vi "CAN_COM.vi"() -> ()   [LabVIEW 2016]
uses:
  <vilib>/Platform/TimedLoop/XDataNode/timing_clust.ctl
  <vilib>/Platform/TimedLoop/XDataNode/nitl_modes.ctl
  <vilib>/Platform/TimedLoop/XDataNode/wakeup.ctl
  <vilib>/platform/TimedLoop/XDataNode/XDataNode.xnode
  <vilib>/Platform/TimedLoop/XDataNode/XDNodeRunTimeDep.lvlib
panel:
  out "MOD_6":bool
  out "MOD_1":bool
  in  "UNLOCK_LEVEL":bool
  in  "Stop RT":bool
  in  "Transmit Frame":T1={"timestamp high"=0, "timestamp low"=0, "identifier"=18, "type"=enum."Data Frame", "info A"=0, "info B"=0, "data length"=8, "data"=[0, 0, 0, 0, 0, 0, 0, 0]} {"identifier" format="%x"; "data" format="%.0x"}
  out "Total Received":u32
  out "Recent Receive":T2={"timestamp high"=0, "timestamp low"=0, "identifier"=0, "type"=enum."Data Frame", "info A"=0, "info B"=0, "data length"=0, "data"=[0, 0, 0, 0, 0, 0, 0, 0]} {"identifier" format="%.0x"; "data" format="%.0x"}
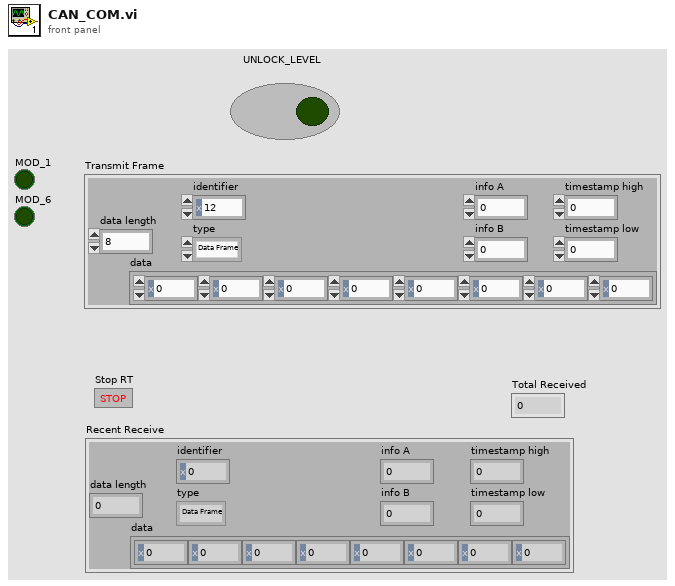
[diagram p1: front panel]
types:
  T1 = cluster{"timestamp high":u32, "timestamp low":u32, "identifier":u32, "type":enum8{"Data Frame", "Remote Frame", "(reserved)", "(reserved) ", "(reserved)  ", "(reserved)   ", "Bus Error", "Transceiver Fault"}, "info A":u8, "info B":u8, "data length":u8, "data":u32[]}
  T2 = cluster{"timestamp high":u32, "timestamp low":u32, "identifier":u32, "type":enum8{"Data Frame", "Remote Frame", "(reserved)", "(reserved) ", "(reserved)  ", "(reserved)   ", "Bus Error", "Transceiver Fault"}, "info A":u8, "info B":u8, "data length":u8, "data":u8[]}
  T3 = typedef "XDNodeRunTimeDep.lvlib/timing_clust.ctl" = cluster{"Expected End [f-1]":u64, "Actual End [f-1]":u64, "Finished Late? [f-1]":bool, "Expected End [i-1]":u64, "Actual End [i-1]":u64, "Finished Late? [i-1]":bool, "Expected Start [i]":u64, "Actual Start [i]":u64, "Expected Start [f]":u64, "Actual Start [f]":u64, "Source Name":string, "Structure Name":string, "Period":i64, "Deadline":i64, "Offset":i64, "Start":i64, "Priority":i32, "Timeout":i32, "Mode":T4, "Wakeup Reason":T5, "Error":errorcluster, "Source Type":string, "Secondary Source Type":string, "Global End Time":u64, "Global Start Time":u64, "Frame Duration":u64, "Iteration Duration":u64, "Assigned CPU":i32, "I/O Scan Engine Mode":u32}
  T4 = typedef "XDNodeRunTimeDep.lvlib/nitl_modes.ctl" = enum32{"No Change", "Process missed periods, maintain original phase", "Discard missed periods, maintain original phase", "Process missed periods, ignore original phase", "Discard missed periods, ignore original phase"}
  T5 = typedef "XDNodeRunTimeDep.lvlib/wakeup.ctl" = enum32{"Normal", "Aborted", "Asynchronous wakeup", "Timing source error", "Timed loop error", "Timeout"}
  T6 = enum8{"Data Frame", "Remote Frame", "(reserved)", "(reserved) ", "(reserved)  ", "(reserved)   ", "Bus Error", "Transceiver Fault"}
  T7 = cluster{"data[0]":u32, "data[1]":u32, "data[2]":u32, "data[3]":u32, "data[4]":u32, "data[5]":u32, "data[6]":u32, "data[7]":u32, "data[8]":u32}
  T8 = cluster{"data[0]":u8, "data[1]":u8, "data[2]":u8, "data[3]":u8, "data[4]":u8, "data[5]":u8, "data[6]":u8, "data[7]":u8, "data[8]":u8}
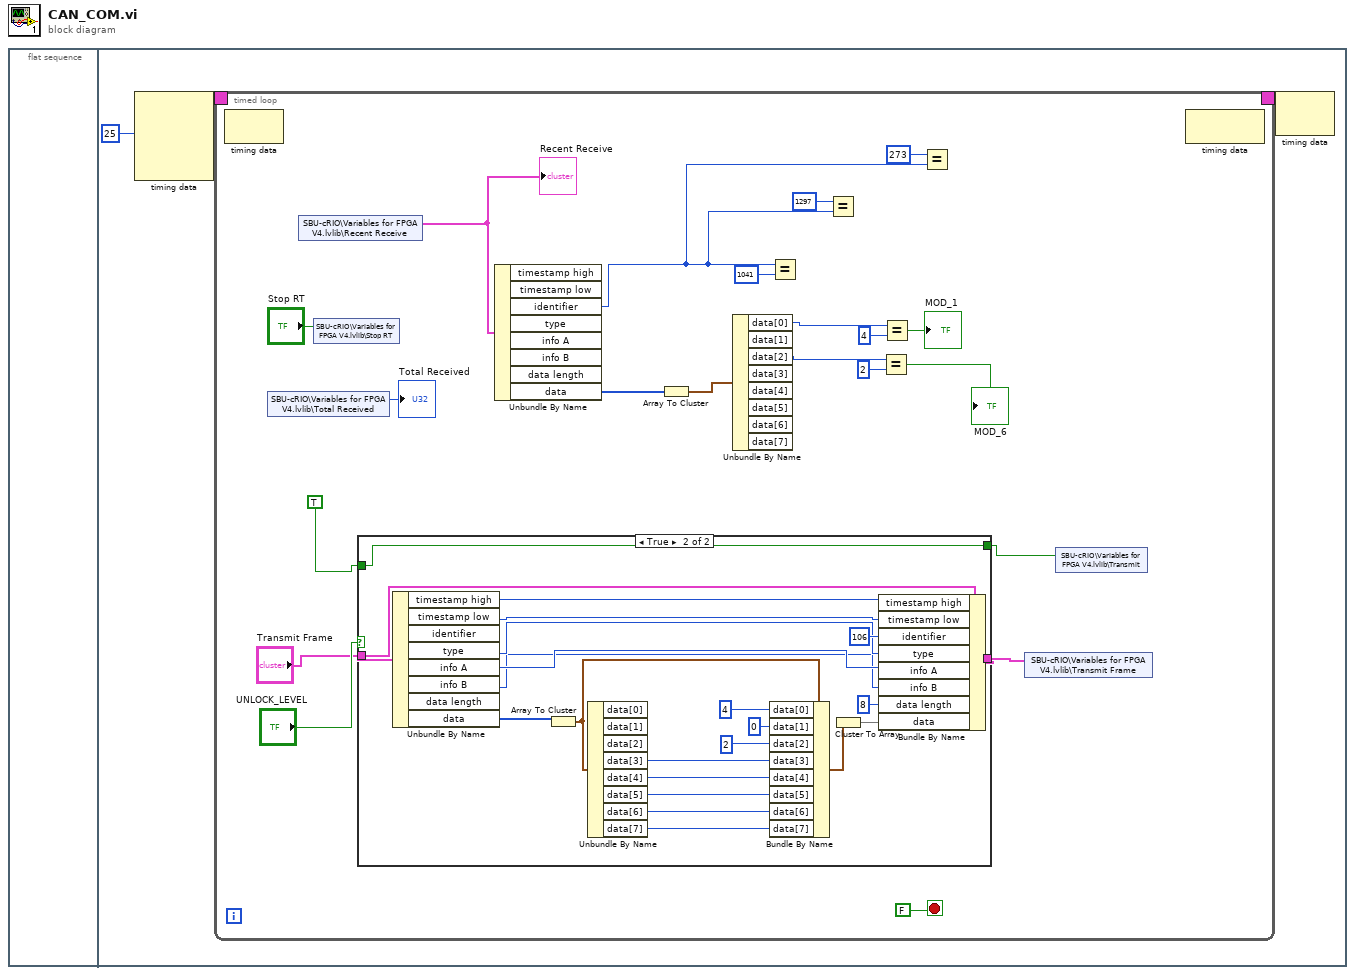
[diagram p0: block diagram]
diagram:
  n1 = flat-sequence {
    frame #0 {
    }
    frame #1 {
      n2 = node-c288(i64 25 ("Period")) -> (w3:T3)  [unwired: 3 in]
      n3 = timed-loop {
        timing: w3 -> [_]
        timing-out: [_] -> w2
        stop <- FALSE stop-if-true
        n4 = node-c288() -> ()  [unwired: 1 in, 1 out]
        n5 = shared-variable "SBU-cRIO\\Variables for FPGA V4.lvlib\\Total Received"() -> (→"Total Received":u32)  [unwired: 1 in, 1 out]
        n6 = shared-variable "SBU-cRIO\\Variables for FPGA V4.lvlib\\Recent Receive"() -> (w18:T2)  [unwired: 1 in, 1 out]
        "Recent Receive" <- w18
        n7 = shared-variable "SBU-cRIO\\Variables for FPGA V4.lvlib\\Stop RT"("Stop RT") -> ()  [unwired: 1 in, 1 out]
        n8 = case shown="True" "UNLOCK_LEVEL" {
          tunnel: "Transmit Frame" -> [w26 w38]
          tunnel: [w26 w39] -> w16
          tunnel: [w25 w34] -> w6
          tunnel: TRUE -> [w25 w34]
          frame False {
          }
          frame True {
            n9 = Unbundle By Name(w38) -> ("timestamp high"=w47:u32, "timestamp low"=w46:u32, "type"=w44:T6, "info A"=w43:u8, "info B"=w42:u8, "data"=w40:u32[])  [unwired: 2 out]
            n10 = Array To Cluster(array=w40) -> (cluster=w37:T7)
            n11 = Unbundle By Name(w37) -> ("data[3]"=w31:u32, "data[4]"=w30:u32, "data[5]"=w29:u32, "data[6]"=w28:u32, "data[7]"=w27:u32)  [unwired: 3 out]
            n12 = Bundle By Name(cluster=w37, "data[0]"=u32 4, "data[1]"=u32 0, "data[2]"=u32 2 ("identifier"), "data[3]"=w31, "data[4]"=w30, "data[5]"=w29, "data[6]"=w28, "data[7]"=w27) -> (w36:T7)
            n13 = Cluster To Array(cluster=w36) -> (array=w41:u32[])
            n14 = Bundle By Name(cluster=w38, "timestamp high"=w47, "timestamp low"=w46, "identifier"=u32 106, "type"=w44, "info A"=w43, "info B"=w42, "data length"=u8 8, "data"=w41) -> (w39:T1)
          }
        }
        n15 = Unbundle By Name(w18) -> ("identifier"=w15:u32, "data"=w17:u8[])  [unwired: 6 out]
        n16 = Array To Cluster(array=w17) -> (cluster=w22:T8)
        n17 = Unbundle By Name(w22) -> ("data[0]"=w13:u8, "data[2]"=w4:u8)  [unwired: 6 out]
        n18 = Equal?(x=w15, y=u32 1041) -> ()  [unwired: 1 out]
        n19 = Equal?(x=u32 1297, y=w15) -> ()  [unwired: 1 out]
        n20 = Equal?(x=w4, y=u8 2) -> (x = y?=→"MOD_6":bool)
        n21 = Equal?(x=w13, y=u8 4) -> (x = y?=→"MOD_1":bool)
        n22 = Equal?(x=u32 273, y=w15) -> ()  [unwired: 1 out]
        n23 = shared-variable "SBU-cRIO\\Variables for FPGA V4.lvlib\\Transmit Frame"(w16) -> ()  [unwired: 1 in, 1 out]
        n24 = shared-variable "SBU-cRIO\\Variables for FPGA V4.lvlib\\Transmit"(w6) -> ()  [unwired: 1 in, 1 out]
        n25 = node-c288() -> ()  [unwired: 1 in, 1 out]
      }
      n26 = node-c288(w2) -> ()  [unwired: 1 out]
    }
  }
